vi "Dual_SVPWM_TimingGen_SGL_gen.vi"(0 "ref_beta":sgl[](array[numeric])=[0.0, 0.0], 5 "Period":i32=1, 7 "ref_max":sgl=0.9999695, 9 "input valid":bool=TRUE, 11 "ref_alpha":sgl[](array[numeric])=[0.0, 0.0]) -> (4 "C_timing":cluster{"ON":u32, "OFF":u32}[](array[cluster]), 6 "B_timing":cluster{"ON":u32, "OFF":u32}[](array[cluster]), 8 "A_timing":cluster{"ON":u32, "OFF":u32}[](array[cluster]), 10 "output valid":bool, 14 "feedback signals":cluster{"ready for input":bool})   [LabVIEW 2015]
doc: "This VI is created by the NI LabVIEW 2015 FPGA IP Builder.\n\nProject: SVPWM_dev.lvproj\nTarget: FPGA Target (sbRIO-9607)/IP Builder\nBuild Specification: Dual_SVPWM_TimingGen_SGL_gen\nDirectives Item: Dual_SVPWM_TimingGen_SGL_src\nTop-Level VI: C:\\LabVIEWPowerElectronicsControl\\SpaceVectorPWM\\dev\\IPBuilder\\Dual_SVPWM_TimingGen_SGL_src.vi\n\nQuick Device Utilization Estimate\n--------------------------------------------\nSlice Registers: 2.4% (2516 out of 106400)\nSlice LUTs: 18.3% (9758 out of 53200)\nDSP48s: 4.1% (9 out of 220)\nBlock RAMs: 0.0% (0 out of 280)\n\nQuick Performance Estimate\n--------------------------------------------\nClock rate (MHz): 46.36\nInitiation interval (cycles): 40\nPipeline type: Not pipelined\nMinimum latency: 39\nMaximum latency: 39"
uses:
  <vilib>/rvi/IPIntegrationNode/IPINode_Typedef/niFpgaIPINodeSupportedFamilies.ctl
  <vilib>/rvi/IPIntegrationNode/IPINode_Utilities/niFpgaIPINodeSimCore.vi
  <vilib>/rvi/IPIntegrationNode/IPINode_Xnode/niFpgaIPINode.xnode
  Dual_SVPWM_TimingGen_SGL_gen Support/IPBlockSimFiles/xsim.dir/m26EC684A_topH/xsimkFE10449CF8BC4E338EB68EE9EBF3D627.dll
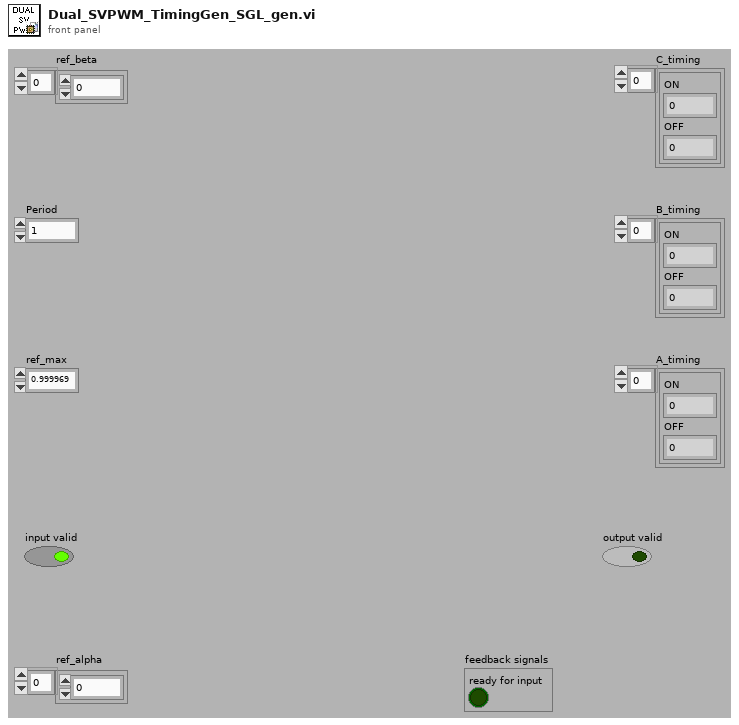
[diagram p1: front panel]
types:
  T1 = cluster{"p_8_C_timing_0_e_0":u32, "p_8_C_timing_0_e_1":u32}
  T2 = cluster{"p_8_C_timing_1_e_0":u32, "p_8_C_timing_1_e_1":u32}
  T3 = cluster{"p_6_B_timing_0_e_0":u32, "p_6_B_timing_0_e_1":u32}
  T4 = cluster{"p_6_B_timing_1_e_0":u32, "p_6_B_timing_1_e_1":u32}
  T5 = cluster{"p_4_A_timing_0_e_0":u32, "p_4_A_timing_0_e_1":u32}
  T6 = cluster{"p_4_A_timing_1_e_0":u32, "p_4_A_timing_1_e_1":u32}
  T7 = cluster{"p_8_C_timing_1_e_0":u32, "p_8_C_timing_1_e_1":u32}[]
  T8 = cluster{"p_6_B_timing_1_e_0":u32, "p_6_B_timing_1_e_1":u32}[]
  T9 = cluster{"p_4_A_timing_1_e_0":u32, "p_4_A_timing_1_e_1":u32}[]
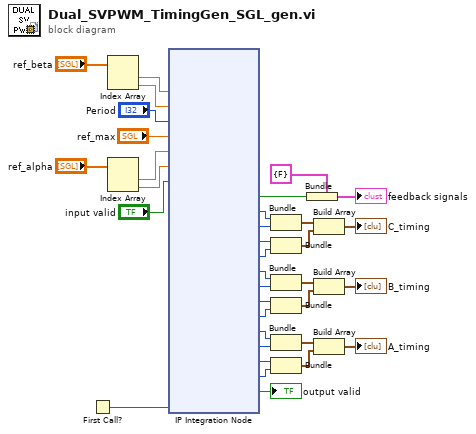
[diagram p0: block diagram]
diagram:
  n1 = First Call?() -> (First Call?: T/F=w35:bool)
  n2 = Index Array(array="ref_beta") -> (element #1=w17:sgl, element #2=w18:sgl)  [unwired: 2 in]
  n3 = Index Array(array="ref_alpha") -> (element #1=w13:sgl, element #2=w14:sgl)  [unwired: 2 in]
  n4 = xnode "IP Integration Node"("p_5_ref_beta_0"=w17, "p_5_ref_beta_1"=w18, "p_2_Period"="Period", "p_1_ref_max"="ref_max", "p_0_ref_alpha_0"=w13, "p_0_ref_alpha_1"=w14, "input_valid"="input valid", "first_call"=w35) -> ("ready_for_input"=w32:bool, "p_8_C_timing_0_e_0"=w9:u32, "p_8_C_timing_0_e_1"=w10:u32, "p_8_C_timing_1_e_0"=w11:u32, "p_8_C_timing_1_e_1"=w12:u32, "p_6_B_timing_0_e_0"=w5:u32, "p_6_B_timing_0_e_1"=w6:u32, "p_6_B_timing_1_e_0"=w7:u32, "p_6_B_timing_1_e_1"=w8:u32, "p_4_A_timing_0_e_0"=w1:u32, "p_4_A_timing_0_e_1"=w2:u32, "p_4_A_timing_1_e_0"=w3:u32, "p_4_A_timing_1_e_1"=w4:u32, "output_valid"=→"output valid":bool)  [unwired: 2 in]
  n5 = Bundle("p_8_C_timing_0_e_0"=w9, "p_8_C_timing_0_e_1"=w10) -> (w25:T1)  [unwired: 1 in]
  n6 = Bundle("p_8_C_timing_1_e_0"=w11, "p_8_C_timing_1_e_1"=w12) -> (w26:T2)  [unwired: 1 in]
  n7 = Bundle("p_6_B_timing_0_e_0"=w5, "p_6_B_timing_0_e_1"=w6) -> (w22:T3)  [unwired: 1 in]
  n8 = Bundle("p_6_B_timing_1_e_0"=w7, "p_6_B_timing_1_e_1"=w8) -> (w23:T4)  [unwired: 1 in]
  n9 = Bundle("p_4_A_timing_0_e_0"=w1, "p_4_A_timing_0_e_1"=w2) -> (w19:T5)  [unwired: 1 in]
  n10 = Bundle("p_4_A_timing_1_e_0"=w3, "p_4_A_timing_1_e_1"=w4) -> (w20:T6)  [unwired: 1 in]
  n11 = Bundle ("Bundle_feedback")(cluster=cluster{"ready for input":bool} {"ready for input"=FALSE}, "ready for input"=w32) -> (→"feedback signals":cluster{"ready for input":bool})
  n12 = Build Array(w25, w26) -> (→"C_timing":T7)
  n13 = Build Array(w22, w23) -> (→"B_timing":T8)
  n14 = Build Array(w19, w20) -> (→"A_timing":T9)
